vi "Filtered Compass.vi"(11 "FPGA Reference In":T1) -> (3 "FPGA Reference Out":T1)   [LabVIEW 2012]
uses:
  FPGA_ref.ctl
  <vilib>/Platform/TimedLoop/XDataNode/timing_clust.ctl
  <vilib>/Platform/TimedLoop/XDataNode/nitl_modes.ctl
  <vilib>/Platform/TimedLoop/XDataNode/wakeup.ctl
  <vilib>/Analysis/coordinate.llb/Angle Units.ctl
  <vilib>/Analysis/coordinate.llb/Angle Range (Degree).ctl
  <vilib>/Analysis/coordinate.llb/Wrap Angle (scalar).vi
  Globals.vi
  <vilib>/platform/TimedLoop/XDataNode/XDataNode.xnode
  <vilib>/Analysis/NI_AAL_Angle.lvlib
  <vilib>/Platform/TimedLoop/XDataNode/XDNodeRunTimeDep.lvlib
  Compass/Compass IO.lvlib
panel:
  out "Gyro Velocities":T2
  out "Filter":dbl(graph)
  out "Gyro":dbl(graph)
  out "Compass":dbl(graph)
  out "Filtered Heading":dbl
  out "Disturbance?":bool
  out "Var":dbl
  out "Finished Late? [i-1]":bool
  out "Iteration Duration":i64
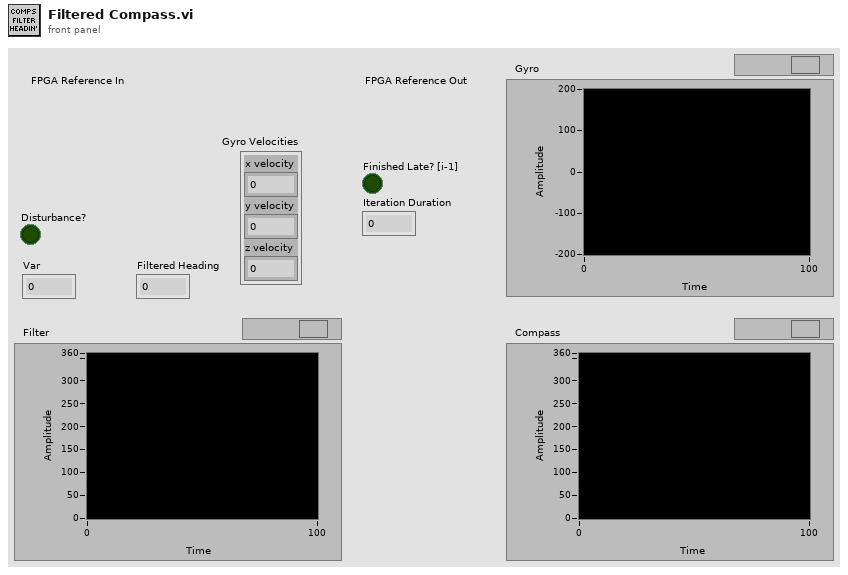
[diagram p1: front panel]
types:
  T1 = typedef "FPGA_ref.ctl" = refnum<k20>
  T2 = cluster{"x velocity":dbl, "y velocity":dbl, "z velocity":dbl}
  T3 = cluster{"FPGA VI Reference":refnum<k20>, "Port Number":u8}
  T4 = typedef "XDNodeRunTimeDep.lvlib/timing_clust.ctl" = cluster{"Expected End [f-1]":u64, "Actual End [f-1]":u64, "Finished Late? [f-1]":bool, "Expected End [i-1]":u64, "Actual End [i-1]":u64, "Finished Late? [i-1]":bool, "Expected Start [i]":u64, "Actual Start [i]":u64, "Expected Start [f]":u64, "Actual Start [f]":u64, "Source Name":string, "Structure Name":string, "Period":i64, "Deadline":i64, "Offset":i64, "Start":i64, "Priority":i32, "Timeout":i32, "Mode":T5, "Wakeup Reason":T6, "Error":errorcluster, "Source Type":string, "Secondary Source Type":string, "Global End Time":u64, "Global Start Time":u64, "Frame Duration":u64, "Iteration Duration":u64, "Assigned CPU":i32, "I/O Scan Engine Mode":u32}
  T5 = typedef "XDNodeRunTimeDep.lvlib/nitl_modes.ctl" = enum32{"No Change", "Process missed periods, maintain original phase", "Discard missed periods, maintain original phase", "Process missed periods, ignore original phase", "Discard missed periods, ignore original phase"}
  T6 = typedef "XDNodeRunTimeDep.lvlib/wakeup.ctl" = enum32{"Normal", "Aborted", "Asynchronous wakeup", "Timing source error", "Timed loop error", "Timeout"}
  T7 = typedef "NI_AAL_Angle.lvlib/Angle Range (Degree).ctl" = u16
  T8 = typedef "NI_AAL_Angle.lvlib/Angle Units.ctl" = i32
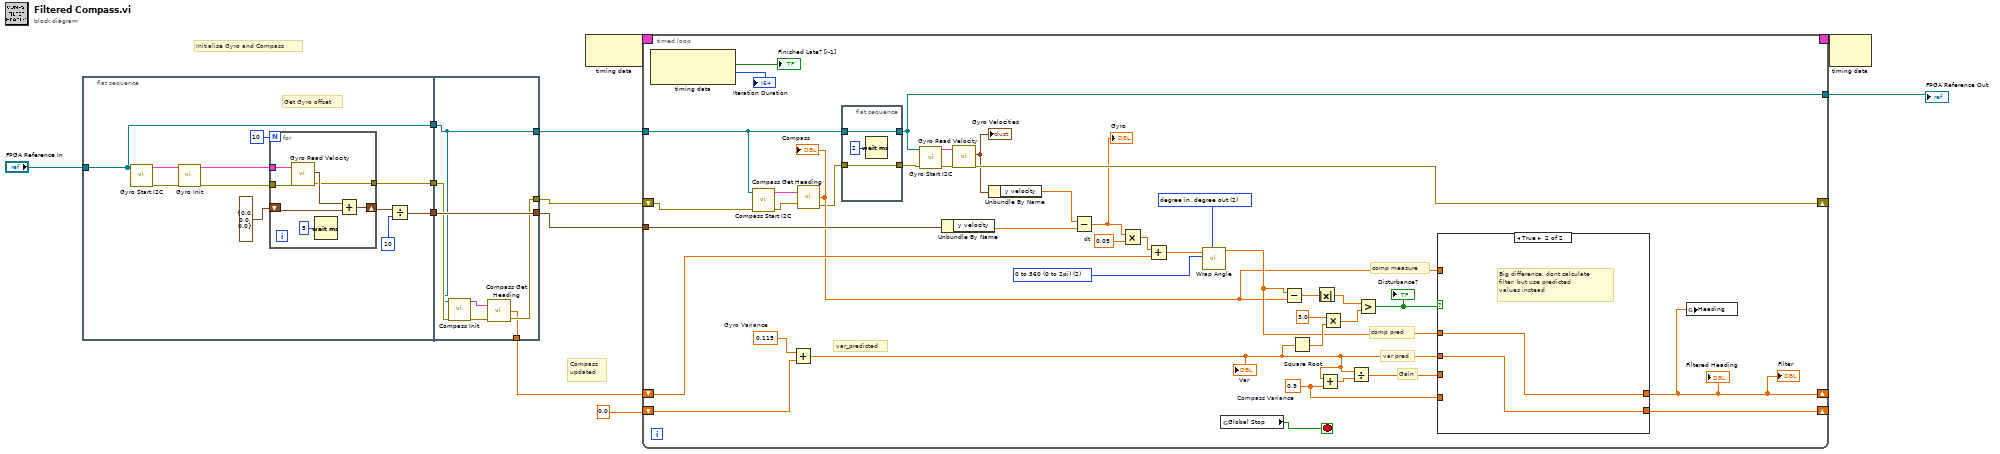
[diagram p0: block diagram]
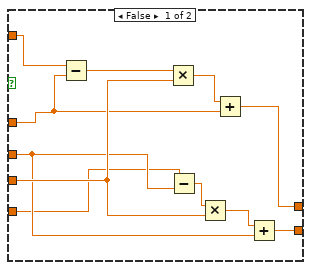
[diagram p2: hidden frame]
diagram:
  # "Initialise Gyro and Compass"
  # "Compass\nupdated"
  n1 = flat-sequence {
    tunnel: [w18] -> w10
    tunnel: [w14] -> w9
    tunnel: [w13] -> w8
    tunnel: "FPGA Reference In" -> [w13]
    tunnel: [w37] -> w7
    tunnel: w10 -> [w37]
    tunnel: w9 -> [w36]
    tunnel: [w33] -> w6
    tunnel: [w32] -> w4
    tunnel: [w31] -> w3
    tunnel: w8 -> [w31]
    frame #0 {
      # "Get Gyro offset"
      n2 = call "Gyro Start I2C.vi"("FPGA Reference In"=w13) -> ("error out"=w16:errorcluster, "I2C Information Out"=w23:T3)  [unwired: 9 in]
      n3 = call "Gyro Init.vi"("error in (no error)"=w16, "I2C Information Out"=w23) -> ("error out"=w15:errorcluster, "FPGA Information Out"=w17:T3)  [unwired: 8 in]
      n4 = for {
        N: 10 -> [_]
        tunnel: w17 -> [w30]
        tunnel: w15 -> [w29]
        shift-right: [w28] -> w20
        shift-left: T2 {"x velocity"=0.0, "y velocity"=0.0, "z velocity"=0.0} -> [w27]
        tunnel: [w24] -> w14
        n5 = call "Gyro Read Velocity.vi"("error in (no error)"=w29, "FPGA Information In"=w30) -> ("error out"=w24:errorcluster, "Gyro Velocities"=w26:T2)  [unwired: 7 in, 1 out]
        n6 = Wait (ms)(milliseconds to wait=u32 5) -> ()  [unwired: 1 out]
        n7 = Add(x=w26, y=w27) -> (x+y=w28:T2)
      }
      n8 = Divide(x=w20, y=10) -> (x/y=w18:T2)
    }
    frame #1 {
      n9 = call "Compass Init.vi"("error in (no error)"=w36, "FPGA VI Reference"=w31) -> ("error out"=w34:errorcluster, "FPGA Information Out"=w35:T3)  [unwired: 6 in]
      n10 = call "Compass Get Heading.vi"("FPGA Information In"=w35, "error in (no error)"=w34) -> ("Heading (deg)"=w32:dbl, "error out"=w33:errorcluster)  [unwired: 1 in]
    }
  }
  n11 = node-c288() -> (w12:T4)  [unwired: 1 in]
  n12 = timed-loop {
    timing: w12 -> [_]
    timing-out: [_] -> w11
    tunnel: w7 -> [w73]
    shift-right: [w77] -> _
    shift-left: w6 -> [w76]
    shift-right: [w61] -> _
    shift-left: 0.0 -> [w68]
    shift-right: [w40] -> _
    shift-left: w4 -> [w70]
    tunnel: w3 -> [w39]
    tunnel: [w38] -> w1
    stop <- w41 stop-if-true
    w53 = 0.9  # Compass Variance
    w66 = T7 2 items=["none", "-180 to 180 (-pi to pi)", "0 to 360 (0 to 2pi)"] ("angle range")
    w67 = T8 2 items=["radian in, radian out", "radian in, degree out", "degree in, degree out", "degree in, radian out"] ("angle units")
    w69 = 0.115  # Gyro Variance
    w71 = 0.05  # dt
    # "comp measure"
    # "var pred"
    # "comp pred"
    # "Gain"
    # "var_predicted"
    n13 = node-c288() -> (→"Finished Late? [i-1]":bool, →"Iteration Duration":i64)  [unwired: 1 in]
    n14 = call "Compass Start I2C.vi"("error in (no error)"=w76, "Refnum in"=w39) -> ("error out"=w44:errorcluster, "FPGA Information Out"=w45:T3)  [unwired: 8 in]
    n15 = Add(x=w69, y=w68) -> (x+y=w55:dbl)
    "Var" <- w55
    n16 = call "Compass Get Heading.vi"("FPGA Information In"=w45, "error in (no error)"=w44) -> ("Heading (deg)"=w59:dbl, "error out"=w42:errorcluster)  [unwired: 1 in]
    "Compass" <- w59
    n17 = flat-sequence {
      tunnel: [w80] -> w43
      tunnel: w42 -> [w80]
      tunnel: w39 -> [w78]
      tunnel: [w78] -> w38
      frame #0 {
        n18 = Wait (ms)(milliseconds to wait=u32 2) -> ()  [unwired: 1 out]
      }
    }
    n19 = call "Gyro Start I2C.vi"("error in"=w43, "FPGA Reference In"=w38) -> ("error out"=w46:errorcluster, "I2C Information Out"=w47:T3)  [unwired: 8 in]
    n20 = Unbundle By Name(w73) -> ("y velocity"=w72:dbl)
    n21 = call "Gyro Read Velocity.vi"("error in (no error)"=w46, "FPGA Information In"=w47) -> ("error out"=w77:errorcluster, "Gyro Velocities"=w75:T2)  [unwired: 7 in, 1 out]
    "Gyro Velocities" <- w75
    n22 = Unbundle By Name(w75) -> ("y velocity"=w74:dbl)
    n23 = Subtract(x=w74, y=w72) -> (x-y=w51:dbl)
    "Gyro" <- w51
    n24 = Multiply(x=w51, y=w71) -> (x*y=w58:dbl)
    n25 = Add(x=w58, y=w70) -> (x+y=w57:dbl)
    n26 = call-poly <vilib>:"Wrap Angle.vi"("angle units"=w67, "angle range"=w66, "angle in"=w57) -> ("angle out"=w60:dbl)  [unwired: 7 in, 1 out]
    n27 = global read "Globals.vi" "Global Stop"() -> (w41:bool)
    n28 = Subtract(x=w60, y=w59) -> (x-y=w65:dbl)
    n29 = Square Root(x=w55) -> (sqrt(x)=w62:dbl)
    n30 = Absolute Value(x=w65) -> (abs(x)=w64:dbl)
    n31 = Add(x=w55, y=w53) -> (x+y=w56:dbl)
    n32 = Multiply(x=3.0, y=w62) -> (x*y=w50:dbl)
    n33 = Divide(x=w55, y=w56) -> (x/y=w54:dbl)
    n34 = Greater?(x=w64, y=w50) -> (0:w52:bool)
    "Disturbance?" <- w52
    n35 = case shown="True" w52 {
      tunnel: w60 -> [w86 w96]
      tunnel: w55 -> [w85 w95]
      tunnel: [w94 w96] -> w40
      tunnel: [w90 w95] -> w61
      tunnel: w59 -> [w93 _]
      tunnel: w54 -> [w88 _]
      tunnel: w53 -> [w84 _]
      frame False {
        n36 = Subtract(x=w93, y=w86) -> (x-y=w91:dbl)
        n37 = Multiply(x=w91, y=w88) -> (x*y=w92:dbl)
        n38 = Subtract(x=w84, y=w85) -> (x-y=w87:dbl)
        n39 = Multiply(x=w87, y=w88) -> (x*y=w89:dbl)
        n40 = Add(x=w92, y=w86) -> (x+y=w94:dbl)
        n41 = Add(x=w89, y=w85) -> (x+y=w90:dbl)
      }
      frame True {
        # "Big difference, dont calculate \nfilter, but use predicted\nvalues instead"
      }
    }
    "Filter" <- w40
    "Filtered Heading" <- w40
    n42 = global write "Globals.vi" "Heading"(w40) -> ()
  }
  "FPGA Reference Out" <- w1
  n43 = node-c288(w11) -> ()  [unwired: 1 out]
